vi "Test_Dwelltime.vi"(8 "error in (no error)":errorcluster, 10 "number of points":i32=4, 11 "Signal Channel":enum16{"Red", "Green"}(ring)) -> (0 "error out":errorcluster, 3 "MaxProj":T1)   [LabVIEW 2020]
doc: "Use this template to create a dialog box with event handling."
uses:
  <vilib>/vision/Image Controls.llb/IMAQ Image.ctl
  Typedefs/Top level VI states.ctl
  Globals/gl_Calibration globals.vi
  Global Variables/gl_Images.vi
  <vilib>/vision/NI_Vision_Development_Module.lvlib
panel:
  in  "Delay":u32=1000
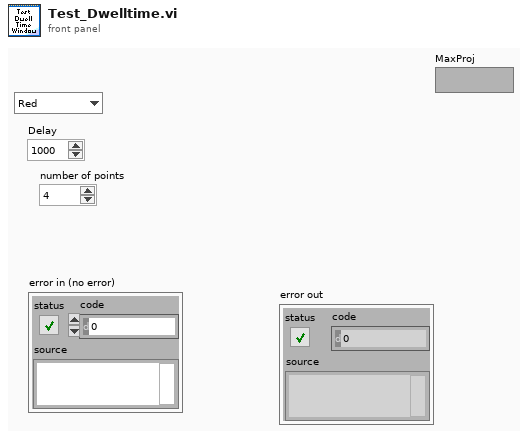
[diagram p1: front panel]
types:
  T1 = typedef "IMAQ Image.ctl" = refnum<image>
  T2 = typedef "Top level VI states.ctl" = enum16{"None", "Initialise UI", "<STACK PROTOCOL STATES>", "AOL Zstack-START", "AOL Zstack-STOP", "Motor Zstack-START", "Motor Zstack-STOP", "<ACQUISITION PROTOCOL STATES> ", "Functional Acquisition-START", "Functional Acquisition-STOP", "Single Plane Acquisition-START", "Single Plane Acquisition-STOP", "Volume Acquisition-START", "Volume Acquisition-STOP", "<LIVE IMAGING PROTOCOL STATES>", "Live Imaging-START", "Live Imaging-STOP", "Live Plane Imaging-START", "Live Plane Imaging-STOP", "Live Volume Imaging-START", "Live Volume Imaging-STOP", "<MOVEMENT CORRECTION PROTOCOL STATES>", "EXIT"}
  T3 = enum32{"Average", "Min", "Max", "Clear  if < ", "Clear  if < or =", "Clear  if =", "Clear  if > or =", "Clear  if >"}
  T4 = typedef "Image Type" = u32
  T5 = typedef "General Scan Parameters.ctl" = cluster{"Field of View":sgl, "Frame Size":u16, "Dwell Time (ms)":dbl, "Wavelength (nm)":dbl, "Zoom":dbl, "AOL Xc":sgl, "AOL Yc":sgl, "AOL Zc":sgl, "AOL Mode":enum16{"Raster", "Structural", "Pointing", "Mini Scan", "Alignment"}, "Imaging Mode":enum16{"Live Imaging", "AOL Zstack", "Motor Zstack", "Functional Imaging"}}
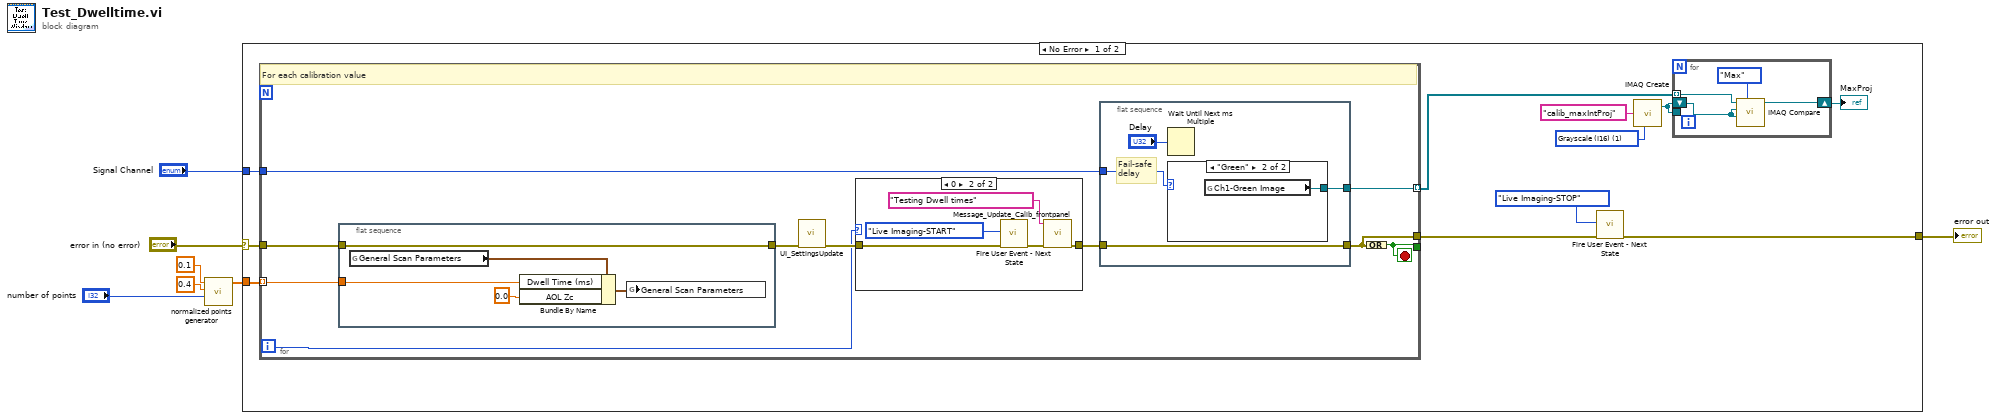
[diagram p0: block diagram]
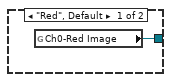
[diagram p3: hidden frame]
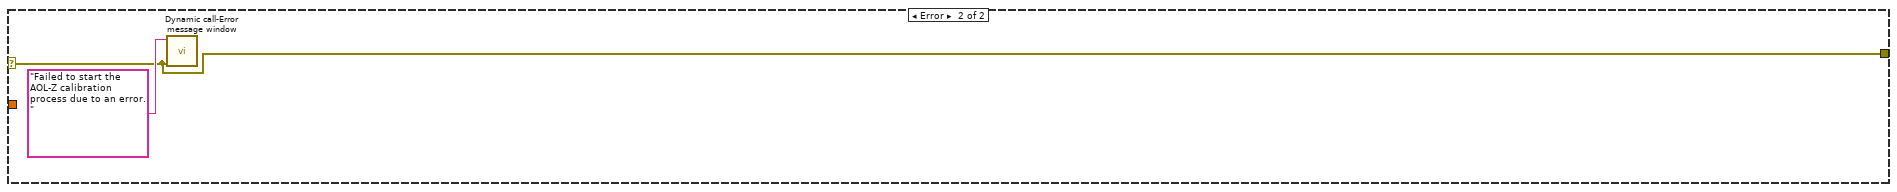
[diagram p4: hidden frame]
diagram:
  n1 = call "normalized points generator.vi"("number of points"="number of points", "maximum"=0.4, "minimum"=0.1) -> ("normalised array"=w5:dbl[])  [unwired: 7 in, 1 out]
  n2 = case shown="No Error" "error in (no error)" {
    selector: "error in (no error)" -> [w17 w50]
    tunnel: w5 -> [w18 _]
    tunnel: [w8 w50] -> w7
    tunnel: "Signal Channel" -> [w16 _]
    frame No Error {
      w13 = T4 1 items=["Grayscale (U8)", "Grayscale (I16)", "Grayscale (SGL)", "Complex (CSG)", "RGB (U32)", "HSL (U32)", "RGB (U64)", "Grayscale (U16)"] ("Image Type")
      n3 = for {
        tunnel: w18 -> [w32] mode=indexing
        tunnel: [w31] -> _
        tunnel: [w26] -> w9
        tunnel: w17 -> [w29]
        tunnel: w16 -> [w25]
        tunnel: [w24] -> w15 mode=indexing
        i -> [w23]
        stop <- w31 stop-if-true
        # "For each calibration value"
        n4 = flat-sequence {
          tunnel: w32 -> [w43]
          tunnel: w29 -> [w39]
          tunnel: [w39] -> w28
          frame #0 {
            n5 = global read "gl_Calibration globals.vi" "General Scan Parameters"() -> (w42:T5)
            n6 = Bundle By Name(cluster=w42, "Dwell Time (ms)"=w43, "AOL Zc"=sgl 0.0 ("AOL Yc")) -> (w41:T5)
            n7 = global write "gl_Calibration globals.vi" "General Scan Parameters"(w41) -> ()
          }
        }
        n8 = call "UI_SettingsUpdate.vi"("error in (no error)"=w28) -> ("error out"=w30:errorcluster)  [unwired: 10 in]
        n9 = case shown="0" w23 {
          tunnel: w30 -> [w33 w38]
          tunnel: [w33 w37] -> w27
          frame 1, Default {
          }
          frame 0 {
            n10 = call "Fire User Event - Next State.vi"("Error In"=w38, "\"UI Handler loop\" case to execute"=Top_level_VI_states."Live Imaging-START" ("\"UI Handler loop\" case to execute")) -> ("Error Out"=w36:errorcluster)  [unwired: 9 in]
            n11 = call "Message_Update_Calib_frontpanel.vi"("error in (no error)"=w36, "Message"="Testing Dwell times") -> ("error out"=w37:errorcluster)  [unwired: 9 in]
          }
        }
        n12 = flat-sequence {
          tunnel: w27 -> [w46]
          tunnel: [w46] -> w26
          tunnel: w25 -> [w45]
          tunnel: [w44] -> w24
          frame #0 {
            # "Fail-safe delay"
            n13 = Wait Until Next ms Multiple(millisecond multiple="Delay") -> ()  [unwired: 1 out]
            n14 = case shown="\"Green\"" w45 {
              tunnel: [w48 w49] -> w44
              frame "Red", Default {
                n15 = global read "gl_Images.vi" "Ch0-Red Image"() -> (w48:T1)
              }
              frame "Green" {
                n16 = global read "gl_Images.vi" "Ch1-Green Image"() -> (w49:T1)
              }
            }
          }
        }
        n17 = Compound Arithmetic op=OR(w26) -> (w31:bool)
      }
      n18 = call "Fire User Event - Next State.vi"("Error In"=w9, "\"UI Handler loop\" case to execute"=Top_level_VI_states."Live Imaging-STOP" ("\"UI Handler loop\" case to execute")) -> ("Error Out"=w8:errorcluster)  [unwired: 9 in]
      n19 = call "IMAQ Create"("Image Name"="calib_maxIntProj", "Image Type"=w13) -> ("New Image"=w12:T1)  [unwired: 3 in, 1 out]
      n20 = for {
        tunnel: w15 -> [w21] mode=indexing
        tunnel: w12 -> [_]
        shift-right: [w20] -> w11
        shift-left: w12 -> [w19]
        n21 = call "IMAQ Compare"("Operator"=T3."Max", "Image Src B"=w19, "Image Dst"=w19, "Image Src A"=w21) -> ("Image Dst Out"=w20:T1)  [unwired: 6 in, 1 out]
      }
      "MaxProj" <- w11
    }
    frame Error {
      n22 = call "Dynamic call-Error message window.vi"("error in (no error)"=w50, "Error Message"="Failed to start the AOL-Z calibration process due to an error.") -> ()  [unwired: 9 in, 1 out]
    }
  }
  "error out" <- w7
